vi "PNGRead.vi"(2 "PNG file path":path=path "/Users/leogallacio/Downloads/N8.png", 7 "Paths error":errorcluster) -> (12 "PNG picture":picture, 13 "PNGRead error":errorcluster, 14 "Pixels colors (uchar)":u32[](array[numeric]), 15 "PNG file path out":path, 16 "Depth":i32, 17 "Width":i16, 18 "Height":i16, 19 "Pixels colors (CLUT)":u8[](array[numeric]))   [LabVIEW 2023]
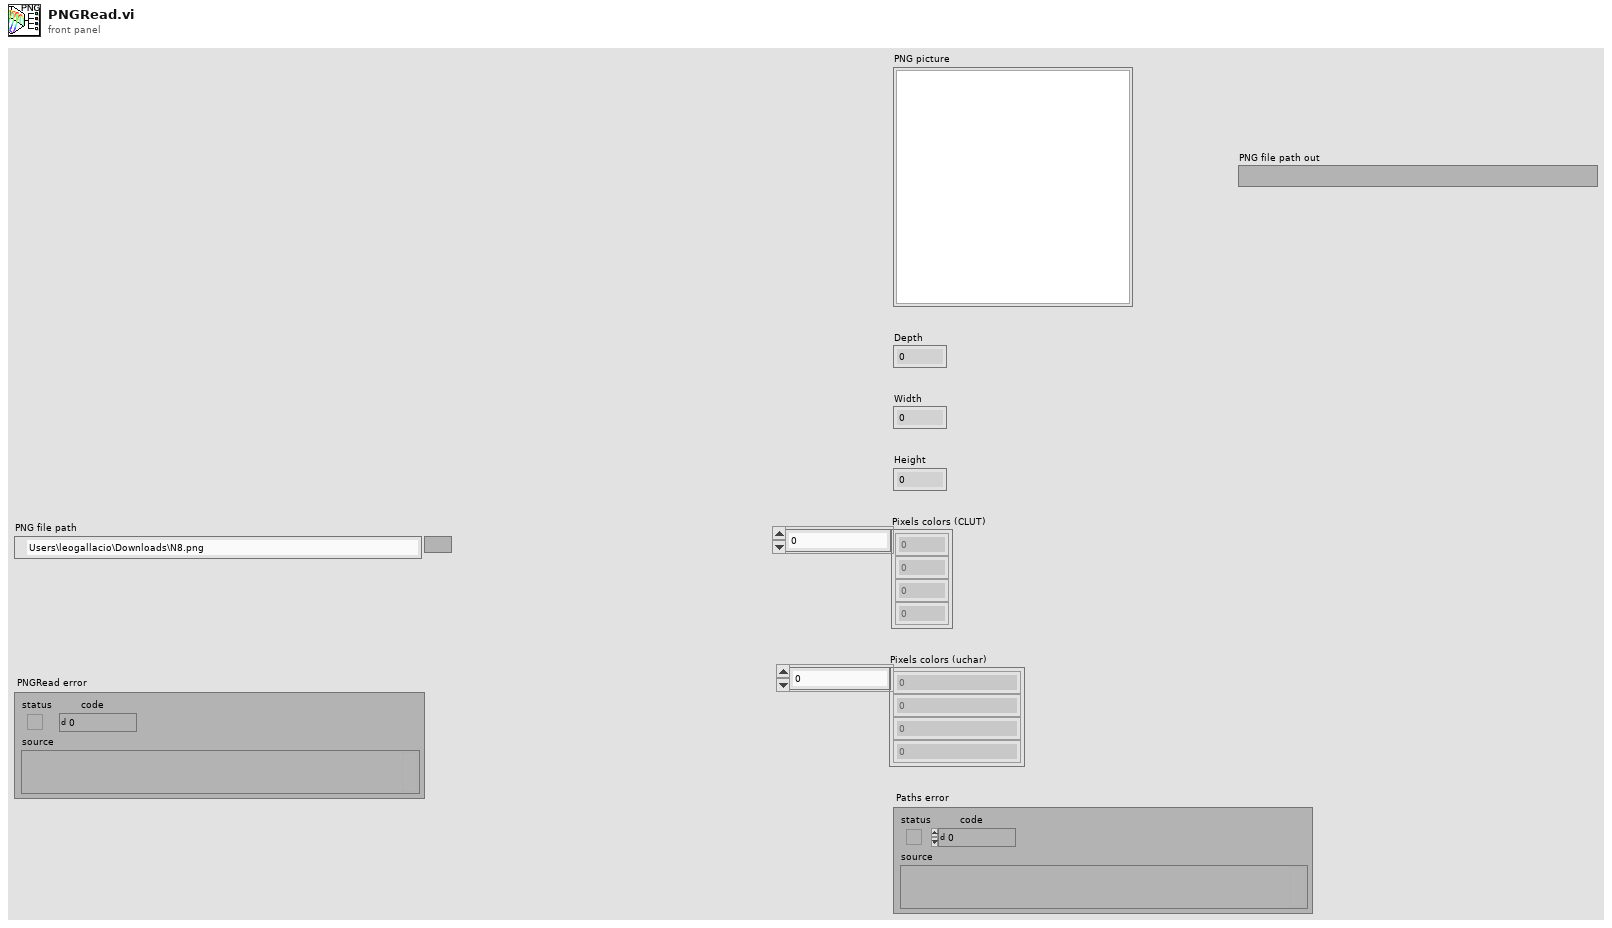
[diagram p1: front panel]
types:
  T1 = typedef "imagedata.ctl" = cluster{"image type":i32, "image depth":i32, "image":u8[], "mask":u8[], "colors":u32[], "Rectangle":cluster{"left":i16, "top":i16, "right":i16, "bottom":i16}}
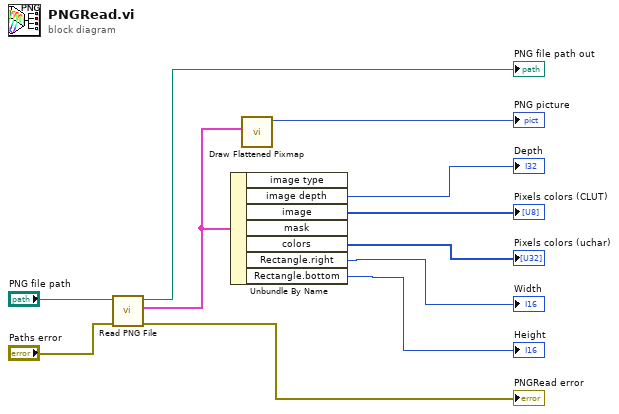
[diagram p0: block diagram]
diagram:
  n1 = call <vilib>:"Read PNG File.vi"("error in (no error)"="Paths error", "path to PNG file"="PNG file path") -> ("error out"=→"PNGRead error":errorcluster, "image data"=w6:T1, "path"=→"PNG file path out":path)  [unwired: 7 in]
  n2 = Unbundle By Name(w6) -> ("image depth"=→"Depth":i32, "image"=→"Pixels colors (CLUT)":u8[], "colors"=→"Pixels colors (uchar)":u32[], "Rectangle.right"=→"Width":i16, "Rectangle.bottom"=→"Height":i16)  [unwired: 2 out]
  n3 = call <vilib>:"Draw Flattened Pixmap.vi"("image data"=w6) -> ("new picture"=→"PNG picture":picture)  [unwired: 8 in]
